vi "Calculate Zstack Positions.vi"(9 "Number of Frames":i32, 10 "XYZ end in":dbl[](array[numeric]), 11 "XYZ start in":dbl[](array[numeric])) -> (2 "Stack Coordinates Out":dbl[][](array[numeric]))   [LabVIEW 2015, in "Automation.lvlib"]
uses:
  Automation.lvlib
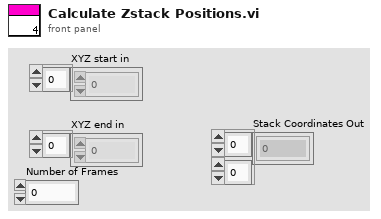
[diagram p1: front panel]
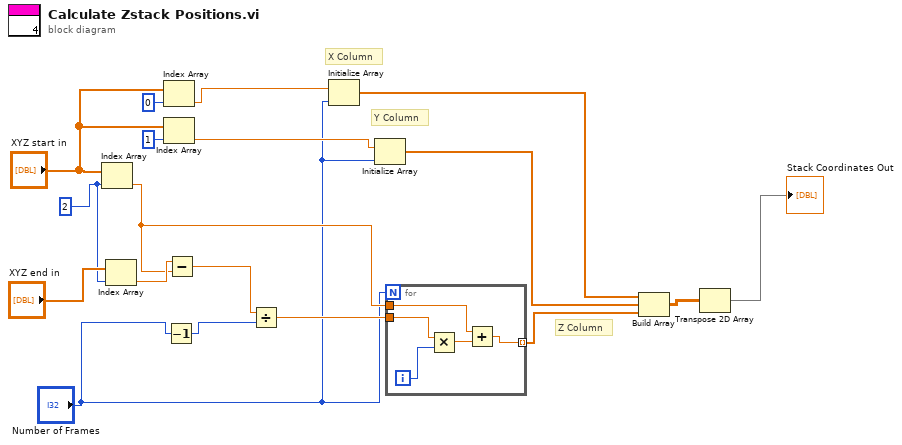
[diagram p0: block diagram]
diagram:
  w16 = 2 ("index")
  # "Z Column"
  # "Y Column"
  # "X Column"
  n1 = Index Array(array="XYZ start in", index=w16) -> (element=w3:dbl)
  n2 = Index Array(array="XYZ end in", index=w16) -> (element=w4:dbl)
  n3 = Index Array(array="XYZ start in", index=0) -> (element=w11:dbl)
  n4 = Index Array(array="XYZ start in", index=1) -> (element=w10:dbl)
  n5 = Decrement(x="Number of Frames") -> (x-1=w1:i32)
  n6 = Subtract(x=w4, y=w3) -> (x-y=w18:dbl)
  n7 = Divide(x=w18, y=w1) -> (x/y=w15:dbl)
  n8 = Initialize Array(w11, "Number of Frames") -> (w7:dbl[])
  n9 = Initialize Array(w10, "Number of Frames") -> (w8:dbl[])
  n10 = for {
    N: "Number of Frames" -> [_]
    tunnel: w15 -> [w23]
    tunnel: [w21] -> w9 mode=indexing
    tunnel: w3 -> [w19]
    i -> [w22]
    n11 = Multiply(x=w23, y=w22) -> (x*y=w20:dbl)
    n12 = Add(x=w19, y=w20) -> (x+y=w21:dbl)
  }
  n13 = Build Array(w7, w8, w9) -> (w6:dbl[][])
  n14 = Transpose 2D Array(2D array=w6) -> (transposed array=→"Stack Coordinates Out":dbl[][])
